vi "subStage_TilingStepSize.vi"(6 "ROI":T1={"Bin"=1, "ROI"={"x offset"=0, "y offset"=0, "x width"=2048, "y width"=2048}} {"ROI"."x offset" min=1 max=512 step=1; "ROI"."y offset" min=1 max=512 step=1; "ROI"."x width" min=1 max=512 step=1; "ROI"."y width" min=1 max=512 step=1; "Bin" items=["1x1"=1, "2x2"=2, "4x4"=4]}, 11 "TI-Ctrl":T2={"Obj"=5, "Cube Bottom"=5, "Cube Top"=1, "PFS-Ctrl"={"PFS IO"=FALSE, "PSF Err"=FALSE, "PSF Pos"=0}, "Z-Ctrl"={"Z-pos"=499.875, "Home"=FALSE, "Sensitivity"=1}, "Condenser"=2, "Lightpath"=enum."EYE"} {"Condenser" items=["A"=1, "DICN2"=2, "- empty 3 -"=3, "- empty 4 -"=4, "- empty 5 -"=5, "- empty 6 -"=6]; "Z-Ctrl"."Sensitivity" min=1 max=3 step=1 scale=1.0..3.0; "PFS-Ctrl"."PSF Pos" scale=0.0..16400.0; "Cube Top" items=["Quad-O"=1, "Quad-R"=2, "empty"=3, "empty"=4, "empty"=5, "DIC"=6]; "Cube Bottom" items=["Cy5"=1, "RFP"=2, "mO2"=3, "empty"=4, "CFP"=5, "GFP"=6]; "Obj" items=["20x/.75 Dry PFS"=1, "40x/1.3 Oil PFS"=2, "60x/1.4 Oil PFS"=3, "- empty 4 -"=4, "- empty 5 -"=5, "- empty 6 -"=6]}) -> (3 "Tiling step size (mm)":dbl[](array[numeric])=[0.22186666666666666, 0.22186666666666666])   [LabVIEW 2015]
panel:
  out "Magnification":dbl=60.0
  # "Calculate step size based on Objective, ROI and binning"
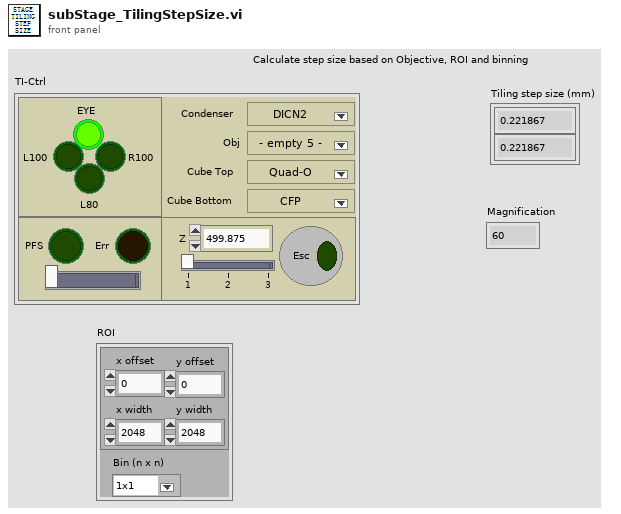
[diagram p1: front panel]
types:
  T1 = cluster{"Bin":u16, "ROI":cluster{"x offset":i32, "y offset":i32, "x width":i32, "y width":i32}}
  T2 = cluster{"Obj":u16, "Cube Bottom":u16, "Cube Top":u16, "PFS-Ctrl":cluster{"PFS IO":bool, "PSF Err":bool, "PSF Pos":u32}, "Z-Ctrl":cluster{"Z-pos":dbl, "Home":bool, "Sensitivity":u8}, "Condenser":u16, "Lightpath":enum32{"EYE", "L100", "R100", "L80"}}
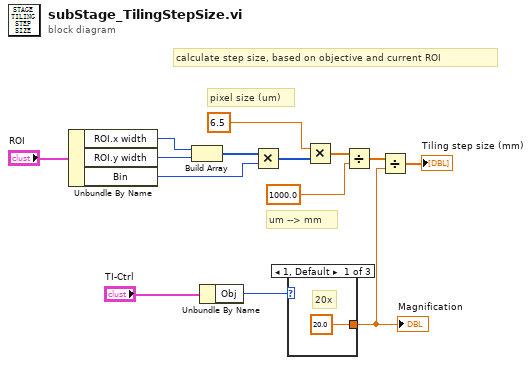
[diagram p0: block diagram]
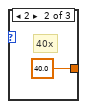
[diagram p2: hidden frame]
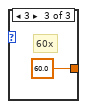
[diagram p3: hidden frame]
diagram:
  # "calculate step size, based on objective and current ROI"
  # "um --> mm"
  # "pixel size (um)"
  n1 = Unbundle By Name("ROI") -> ("ROI.x width"=w10:i32, "ROI.y width"=w9:i32, "Bin"=w3:u16)
  n2 = Build Array(w10, w9) -> (w8:i32[])
  n3 = Unbundle By Name("TI-Ctrl") -> ("Obj"=w1:u16)
  n4 = Multiply(x=w8, y=w3) -> (x*y=w7:i32[])
  n5 = case shown="1, Default" w1 {
    tunnel: [20.0 ("y") 40.0 ("y") 60.0 ("y")] -> w5
    frame 1, Default {
      # "20x"
    }
    frame 2 {
      # "40x"
    }
    frame 3 {
      # "60x"
    }
  }
  "Magnification" <- w5
  n6 = Multiply(x=6.5 ("y"), y=w7) -> (x*y=w13:dbl[])
  n7 = Divide(x=w13, y=1000.0) -> (x/y=w11:dbl[])
  n8 = Divide(x=w11, y=w5) -> (x/y=→"Tiling step size (mm)":dbl[])
